vi "TRAJECTORY_EXECUTE_SWERVE_REVERSE.vi"(8 "Init":bool, 11 "Gyro Heading":dbl) -> (0 "AtReference":bool, 1 "Omega Velocity Target":dbl, 2 "Y Velocity Target":dbl, 3 "X Velocoty Target":dbl, 4 "Error Pose":T1 {"ROTATION"."SIN" format="%13.4f"; "ROTATION"."COS" format="%13.4f"; "ROTATION"."VALUE" format="%13.4f"; "TRANSLATION"."Y" format="%14.3f"; "TRANSLATION"."X" format="%14.3f"})   [LabVIEW 2019]
uses:
  <vilib>/Rock Robotics/WPI/ThirdParty/JAS_Junk/TrajLib/POSE2D.ctl
  <vilib>/Rock Robotics/WPI/ThirdParty/JAS_Junk/TrajLib/TRANSLATION2D.ctl
  <vilib>/Rock Robotics/WPI/ThirdParty/JAS_Junk/TrajLib/ROTATION2D.ctl
  <vilib>/Rock Robotics/WPI/ThirdParty/JAS_Junk/TrajLib/Translation_Create.vi
  <vilib>/Rock Robotics/WPI/ThirdParty/JAS_Junk/TrajLib/Transform_Create_PosePose.vi
  <vilib>/Rock Robotics/WPI/ThirdParty/JAS_Junk/TrajLib/Pose_New_TRRO.vi
  <vilib>/Rock Robotics/WPI/ThirdParty/JAS_Junk/TrajLib/Rotation_UnaryMinus.vi
  <vilib>/Rock Robotics/WPI/ThirdParty/JAS_Junk/TrajLib/Translation_RotateBy.vi
  <vilib>/Rock Robotics/WPI/ThirdParty/JAS_Junk/TrajLib/Translation_Minus.vi
  <vilib>/Rock Robotics/WPI/ThirdParty/JAS_Junk/TrajLib/Rotation_Minus.vi
  <vilib>/Rock Robotics/WPI/ThirdParty/JAS_Junk/TrajLib/Rotation_RotateBy.vi
  <vilib>/Rock Robotics/WPI/ThirdParty/JAS_Junk/TrajLib/Rotation_CreateXY.vi
  <vilib>/Rock Robotics/WPI/ThirdParty/JAS_Junk/TrajLib/Util_CalcDist.vi
  <vilib>/Rock Robotics/WPI/ThirdParty/JAS_Junk/TrajLib/Trajectory_Library.lvlib
  Secret_Control_Library_Protected/Secret_Control_Library_Protected.lvlib
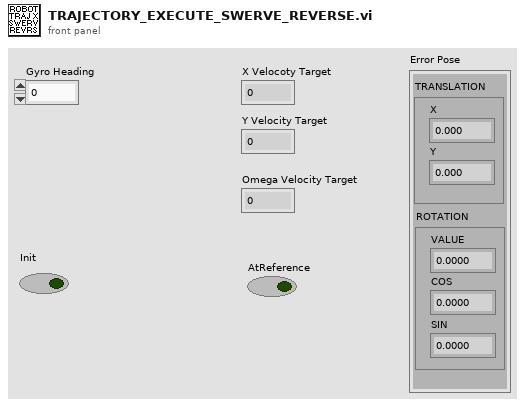
[diagram p1: front panel]
types:
  T1 = typedef "Trajectory_Library.lvlib/POSE2D.ctl" = cluster{"TRANSLATION":T2, "ROTATION":T3}
  T2 = typedef "Trajectory_Library.lvlib/TRANSLATION2D.ctl" = cluster{"X":dbl, "Y":dbl}
  T3 = typedef "Trajectory_Library.lvlib/ROTATION2D.ctl" = cluster{"VALUE":dbl, "COS":dbl, "SIN":dbl}
  T4 = typedef "Trajectory_Library.lvlib/SWERVE_DRIVE_ODOMETRY.ctl" = cluster{"POSE":T1, "GyroOffset":T3, "PreviousAngle":T3, "PrevTime":dbl}
  T5 = typedef "Trajectory_Library.lvlib/SWERVE_DRIVE_KINEMATICS.ctl" = cluster{"NumModules":i32, "InverseKinematics":T6, "ForwardKinematics":T6, "Modules":T2[], "PrevCoR":T2}
  T6 = typedef "NI_Matrix.lvlib/RealMatrix.ctl" = dbl[][]
  T7 = typedef "Trajectory_Library.lvlib/SWERVE_DRIVE_MODULE_STATE.ctl" = cluster{"Speed":dbl, "Angle":T3}
  T8 = typedef "Trajectory_Library.lvlib/TRAJECTORY.ctl" = cluster{"TotalTImeSecs":dbl, "States":T9[]}
  T9 = typedef "Trajectory_Library.lvlib/TRAJ_STATE.ctl" = cluster{"TimeSeconds":dbl, "Velocity":dbl, "Acceleration":dbl, "POSE":T1, "Curvature":dbl}
  T10 = typedef "Trajectory_Library.lvlib/CHASSIS_SPEEDS.ctl" = cluster{"vX":dbl, "vY":dbl, "vOmega":dbl}
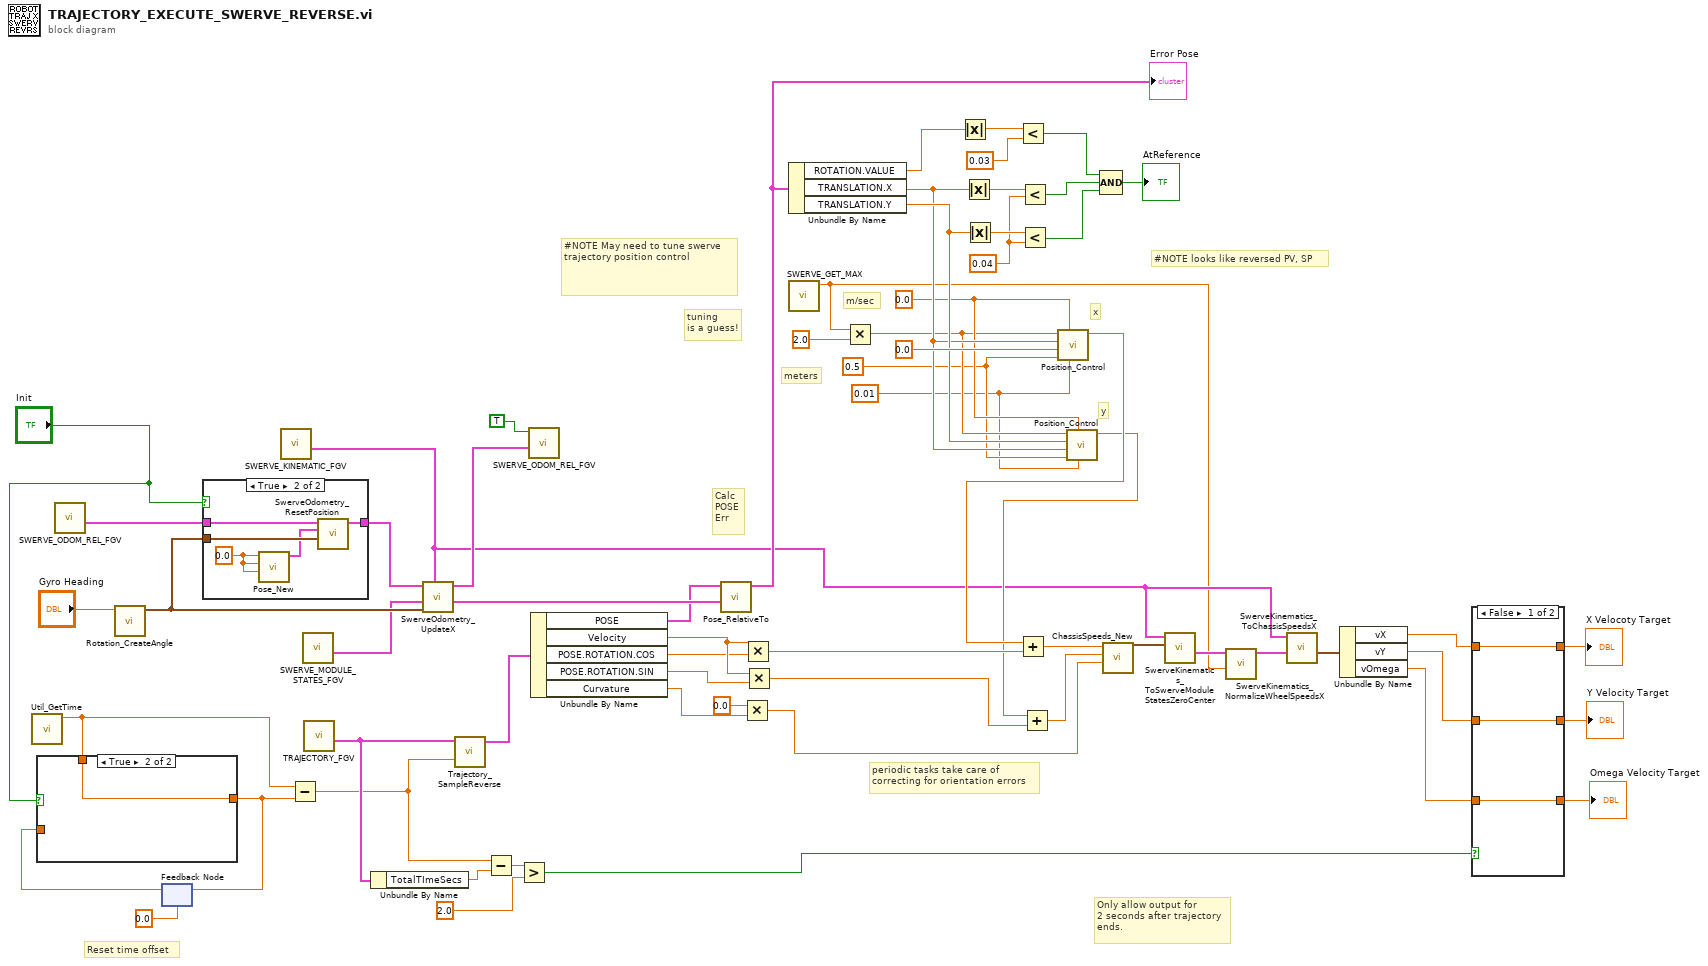
[diagram p0: block diagram]
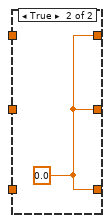
[diagram p3: hidden frame]
diagram:
  w5 = 0.5 ("ErrThreshold")
  w4 = 0.01 ("ErrThreshold")
  w9 = 0.0 ("MinOutput")
  w30 = 0.04
  # "Calc\nPOSE\nErr"
  # "#NOTE looks like reversed PV, SP"
  # "#NOTE May need to tune swerve trajectory position control"
  # "tuning\nis a guess!"
  # "m/sec"
  # "meters"
  # "y"
  # "x"
  # "periodic tasks take care of\ncorrecting for orientation errors"
  # "Only allow output for\n2 seconds after trajectory\nends."
  # "Reset time offset"
  n1 = call <vilib>:"Util_GetTime.vi"() -> ("FPGA_Time_Seconds"=w2:dbl)  [unwired: 10 in, 1 out]
  n2 = call "SWERVE_ODOM_REL_FGV.vi"() -> ("out SWERVE_DRIVE_ODOMETRY"=w52:T4)  [unwired: 11 in]
  n3 = call <vilib>:"Rotation_CreateAngle.vi"("Angle"="Gyro Heading") -> ("ROTATION"=w50:T3)  [unwired: 10 in]
  n4 = feedback #1(0.0 ("TIME")) -> (w63:dbl)
  n5 = case shown="True" "Init" {
    tunnel: [w65 w66] -> w62
    tunnel: w63 -> [w65 _]
    tunnel: w2 -> [_ w66]
    frame False {
    }
    frame True {
    }
  }
  n6 = feedback-in #1(w62) -> ()
  n7 = case shown="True" "Init" {
    tunnel: w52 -> [w67 w72]
    tunnel: [w67 w71] -> w51
    tunnel: w50 -> [_ w70]
    frame False {
    }
    frame True {
      w69 = 0.0 ("X")
      n8 = call <vilib>:"Pose_New.vi"("Heading"=w69, "Y"=w69, "X"=w69) -> ("out POSe"=w68:T1)  [unwired: 8 in]
      n9 = call <vilib>:"SwerveOdometry_ResetPosition.vi"("gyroAngle"=w70, "Pose"=w68, "in SWERVE_DRIVE_ODOMETRY"=w72) -> ("out SWERVE_DRIVE_ODOMETRY"=w71:T4)  [unwired: 8 in]
    }
  }
  n10 = call "SWERVE_KINEMATIC_FGV.vi"() -> ("out SWERVE_DRIVE_KINEMATICS"=w13:T5)  [unwired: 11 in]
  n11 = Subtract(x=w2, y=w62) -> (x-y=w59:dbl)
  n12 = call "SWERVE_MODULE_STATES_FGV.vi"() -> ("out Current Module States"=w47:T7[])  [unwired: 11 in]
  n13 = call "TRAJECTORY_FGV.vi"() -> ("outTRAJECTORY"=w61:T8)  [unwired: 11 in]
  n14 = Unbundle By Name(w61) -> ("TotalTImeSecs"=w60:dbl)
  n15 = call <vilib>:"SwerveOdometry_UpdateX.vi"("SWERVE_DRIVE_KINEMATICS"=w13, "gyroAngle"=w50, "module States"=w47, "in SWERVE_DRIVE_ODOMETRY"=w51) -> ("robot POSE"=w46:T1, "out SWERVE_DRIVE_ODOMETRY"=w48:T4)  [unwired: 6 in]
  n16 = call <vilib>:"Trajectory_SampleReverse.vi"("Time"=w59, "InputTRAJECTORY"=w61) -> ("OutputTRAJ_STATE"=w45:T9)  [unwired: 9 in]
  n17 = Subtract(x=w59, y=w60) -> (x-y=w58:dbl)
  n18 = Greater?(x=w58, y=2.0) -> (0:w56:bool)
  n19 = call "SWERVE_ODOM_REL_FGV.vi"("in SWERVE_DRIVE_ODOMETRY"=w48, "WRITE"=TRUE) -> ()  [unwired: 9 in, 1 out]
  n20 = Unbundle By Name(w45) -> ("POSE"=w44:T1, "Velocity"=w42:dbl, "POSE.ROTATION.COS"=w41:dbl, "POSE.ROTATION.SIN"=w40:dbl, "Curvature"=w39:dbl)
  n21 = call <vilib>:"Pose_RelativeTo.vi"("other POSE"=w46, "in POSE"=w44) -> ("out POSE"=w43:T1)  [unwired: 9 in]
  "Error Pose" <- w43
  n22 = Multiply(x=0.0, y=w39) -> (x*y=w18:dbl)
  n23 = Multiply(x=w42, y=w41) -> (x*y=w36:dbl)
  n24 = Multiply(x=w42, y=w40) -> (x*y=w37:dbl)
  n25 = Unbundle By Name(w43) -> ("ROTATION.VALUE"=w35:dbl, "TRANSLATION.X"=w23:dbl, "TRANSLATION.Y"=w24:dbl)
  n26 = call "SWERVE_GET_MAX.vi"() -> ("Max Wheel Vel (Meter/Sec)"=w8:dbl)  [unwired: 10 in, 1 out]
  n27 = Multiply(x=w8, y=2.0) -> (x*y=w6:dbl)
  n28 = Absolute Value(x=w35) -> (abs(x)=w34:dbl)
  n29 = Absolute Value(x=w23) -> (abs(x)=w33:dbl)
  n30 = Absolute Value(x=w24) -> (abs(x)=w32:dbl)
  n31 = Less?(x=w34, y=0.03) -> (x < y?=w29:bool)
  n32 = Less?(x=w33, y=w30) -> (x < y?=w28:bool)
  n33 = Less?(x=w32, y=w30) -> (x < y?=w27:bool)
  n34 = call "Position_Control.vi"("ErrDeadband"=w4, "MinOutput"=w9, "ErrThreshold"=w5, "CurrentPosition"=0.0, "TargetPosition"=w23, "MaxOutput"=w6) -> ("Output"=w22:dbl)  [unwired: 3 in, 2 out]
  n35 = Add(x=w22, y=w36) -> (x+y=w20:dbl)
  n36 = call "Position_Control.vi"("ErrDeadband"=w4, "MinOutput"=w9, "ErrThreshold"=w5, "CurrentPosition"=w23, "TargetPosition"=w24, "MaxOutput"=w6) -> ("Output"=w21:dbl)  [unwired: 3 in, 2 out]
  n37 = Add(x=w21, y=w37) -> (x+y=w19:dbl)
  n38 = Compound Arithmetic op=AND(w29, w28, w27) -> (→"AtReference":bool)
  n39 = call <vilib>:"ChassisSpeeds_New.vi"("vAngular"=w18, "vY"=w19, "vX"=w20) -> ("CHASSIS"=w17:T10)  [unwired: 8 in]
  n40 = call <vilib>:"SwerveKinematics_ToSwerveModuleStatesZeroCenter.vi"("ChassisSpeeds"=w17, "in SWERVE_DRIVE_KINEMATICS"=w13) -> ("ModuleStates"=w16:T7[])  [unwired: 8 in, 1 out]
  n41 = call <vilib>:"SwerveKinematics_NormalizeWheelSpeedsX.vi"("AttainableMaxSpeed"=w8, "in WheelStates"=w16) -> ("out WheelStates"=w14:T7[])  [unwired: 9 in]
  n42 = call <vilib>:"SwerveKinematics_ToChassisSpeedsX.vi"("WheelStates"=w14, "in SWERVE_DRIVE_KINEMATICS"=w13) -> ("Chassis Speed"=w15:T10)  [unwired: 9 in]
  n43 = Unbundle By Name(w15) -> ("vX"=w12:dbl, "vY"=w11:dbl, "vOmega"=w10:dbl)
  n44 = case shown="False" w56 {
    tunnel: [w74 w76] -> w55
    tunnel: [w73 w76] -> w54
    tunnel: [w75 w76] -> w38
    tunnel: w10 -> [w75 _]
    tunnel: w12 -> [w74 _]
    tunnel: w11 -> [w73 _]
    frame False {
    }
    frame True {
      w76 = 0.0
    }
  }
  "X Velocoty Target" <- w55
  "Y Velocity Target" <- w54
  "Omega Velocity Target" <- w38
